vi "Analytical.vi"() -> ()   [LabVIEW 2013]
panel:
  in  "Tar Sample IL SP":dbl
  in  "XV-741 ILock":bool
  out "TI-741":dbl
  out "HT-741 Tar Sampler":dynamicdata(graph)
  in  "HT-741 SP":dbl
  in  "Auto 8":bool=TRUE
  out "TS2":bool
  out "TS4":bool
  out "TS3":bool
  out "TS1":bool
  in  "XV-741":bool
  out "TI-742":dbl format="%.1f"
  out "TI-743":dbl format="%.1f"
  out "TI-744":dbl format="%.1f"
  out "TI-745":dbl format="%.1f"
  out "TI-746":dbl format="%.1f"
  out "TS5":bool
  out "PI-701":dbl
  out "Acetylene":dbl
  out "O2":dbl
  out "Ar":dbl
  out "Propylene":dbl
  out "Ethylene":dbl
  out "N2":dbl
  out "Gas produced":dbl
  out "H2":dbl
  out "CH4":dbl
  out "CO":dbl
  out "% Conversion":dbl
  out "Propane":dbl
  out "Ethane":dbl
  out "Norm. CH4":dbl
  out "CO2":dbl
  out "H2:CO":dbl
  out "NDIR":dynamicdata(graph)
  in  "XV-701":bool
  out "NDIR CO2":dbl
  out "NDIR CH4":dbl
  out "NDIR CO":dbl
  out "XV-201 IL 2":bool
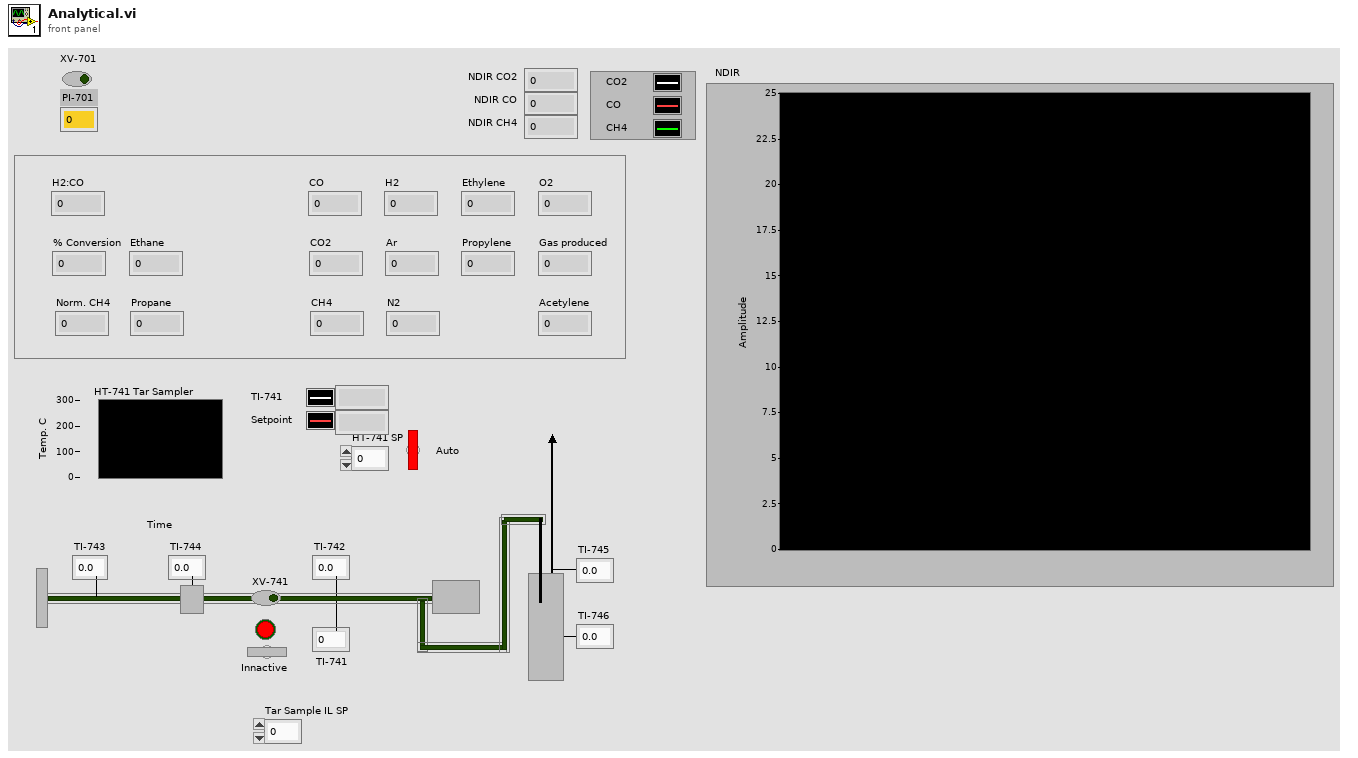
[diagram p1: front panel]
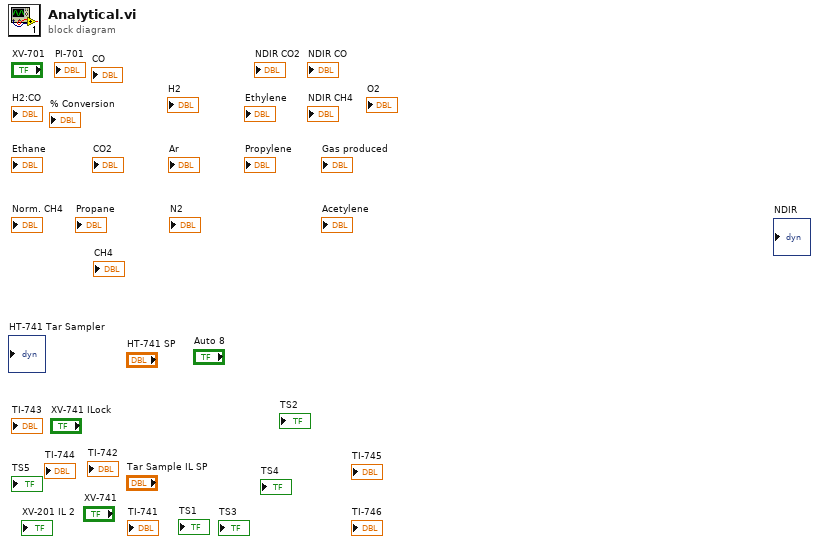
[diagram p0: block diagram]
diagram:
